vi "SVDForPointSetCovarainces.vi"(8 "error in (no error)":errorcluster, 11 "Covariance A & B":T1) -> (0 "error out":errorcluster, 1 "V":T1, 2 "D":T1, 3 "U":T1)   [LabVIEW 2020, in "ar.lvlib"]
uses:
  ar.lvlib
  <vilib>/Analysis/Matrix/Datatypes/RealMatrix.ctl
  <vilib>/Analysis/7linalg.llb/SVD Option.ctl
  <vilib>/Analysis/7linalg.llb/Real SVD Decomposition.vi
  <vilib>/Analysis/NI_AALPro.lvlib
  <vilib>/Analysis/Matrix/NI_Matrix.lvlib
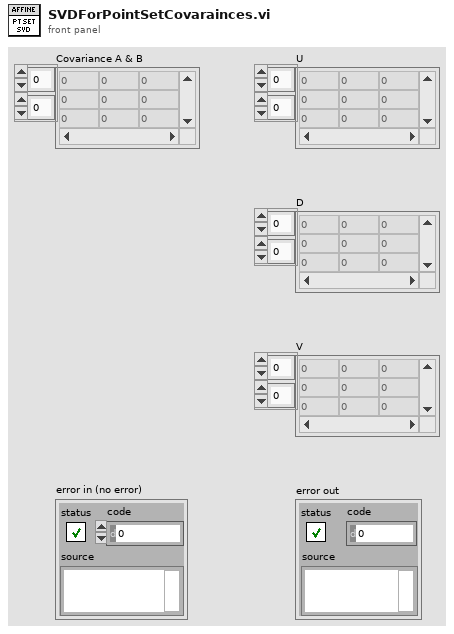
[diagram p1: front panel]
types:
  T1 = typedef "NI_Matrix.lvlib/RealMatrix.ctl" = dbl[][]
  T2 = typedef "NI_AALPro.lvlib/SVD Option.ctl" = u16
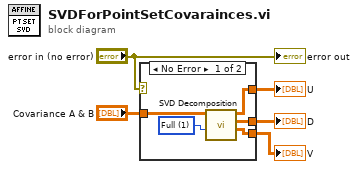
[diagram p0: block diagram]
diagram:
  n1 = case shown="No Error" "error in (no error)" {
    tunnel: [w10 _] -> w5
    tunnel: [w9 _] -> w4
    tunnel: "Covariance A & B" -> [w8 _]
    tunnel: [w7 _] -> w2
    frame No Error {
      w6 = T2 1 items=["Thin", "Full"] ("SVD option")
      n2 = call-poly <vilib>:"SVD Decomposition.vi"("SVD option"=w6, "A"=w8) -> ("Matrix V"=w7:T1, "Matrix S"=w10:T1, "Matrix U"=w9:T1)  [unwired: 5 in, 2 out]
    }
    frame Error {
    }
  }
  "D" <- w5
  "U" <- w4
  "V" <- w2
  "error out" <- "error in (no error)"
